vi "new Maze.vi"(8 "error in (no error)":errorcluster) -> (0 "error out":errorcluster, 3 "Maze* out":refnum<data-value>)   [LabVIEW 2016, in "Maze.lvclass"]
uses:
  Maze.lvclass
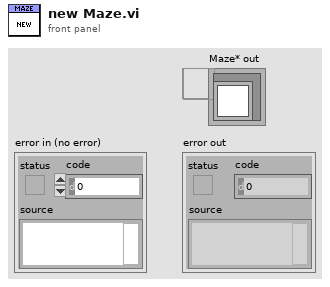
[diagram p1: front panel]
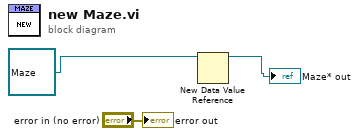
[diagram p0: block diagram]
diagram:
  n1 = New Data Value Reference(data value=refnum<class "Maze.lvclass"> refnum ("Maze in")) -> (data value reference=→"Maze* out":refnum<data-value>)  [unwired: 1 in, 1 out]
  "error out" <- "error in (no error)"
